vi "Power Output PWM Calibration Warning.vi"(8 "error in (no error)":errorcluster={"status"=FALSE, "code"=0, "source"="WinUtil Master.vi"}, 11 "Message (\"\")":string="The PWM must be calibrated with each execution of this test step.  Spartan always records the instrument calibration state when test sequences are executed.\n\nPlease select one of the following options:\n\n    Calibrate  -  run a calibration on the instrument now\n    Ignore  -  continue without calibration\n    Abort  -  abort this test step\n    Abort All  -  abort the entire sequence") -> (0 "error out":errorcluster={"status"=FALSE, "code"=0, "source"="WinUtil Master.vi"}, 3 "Choice":T1=enum."Calibrate")   [LabVIEW 2011]
uses:
  TypeDefs/Power Output Dialog Response.ctl
panel:
  in  "Abort All":bool
  in  "Abort":bool
  in  "Ignore":bool
  in  "Calibrate":bool
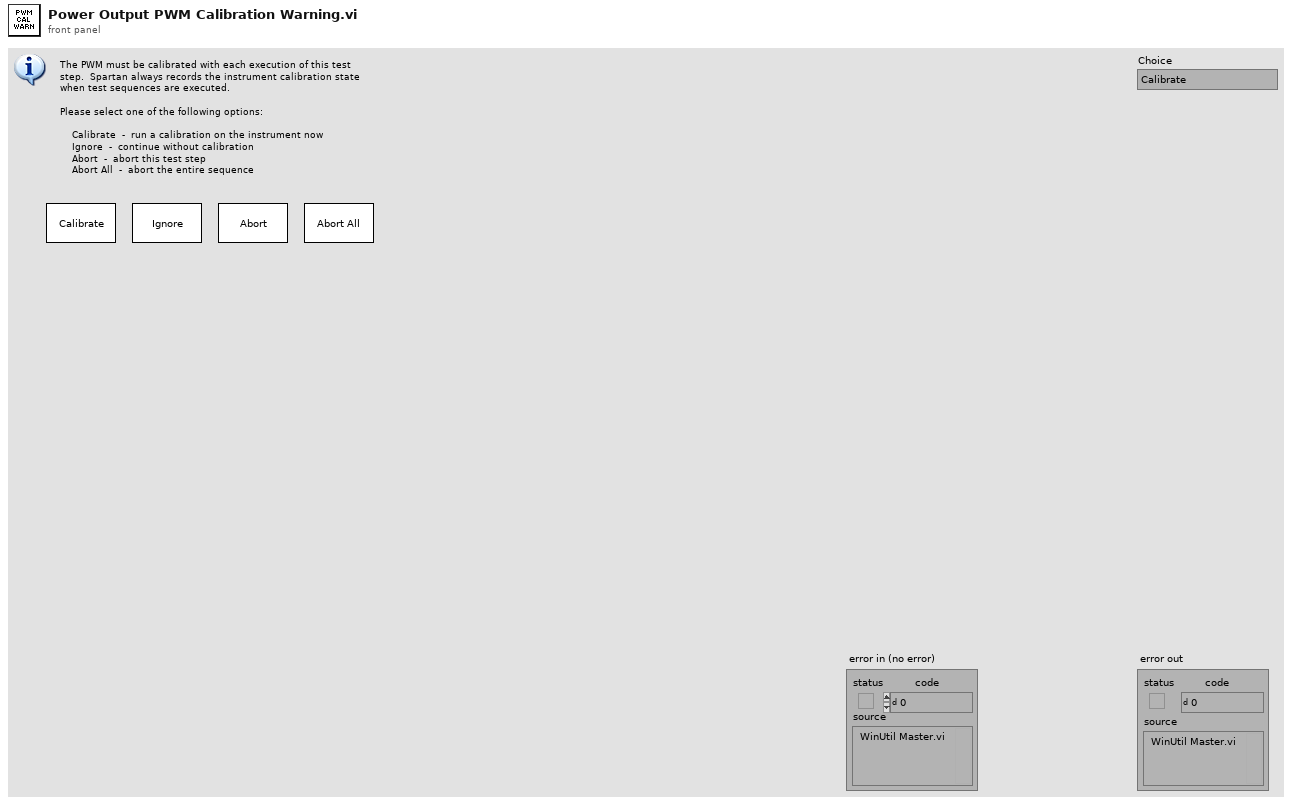
[diagram p1: front panel]
types:
  T1 = typedef "Power Output Dialog Response.ctl" = enum16{"Continue", "Calibrate", "Ignore", "Abort", "Abort All"}
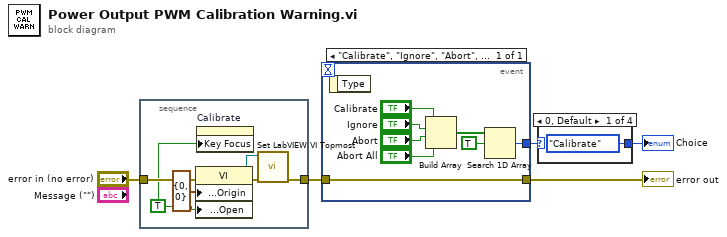
[diagram p0: block diagram]
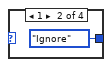
[diagram p2: hidden frame]
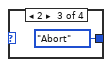
[diagram p3: hidden frame]
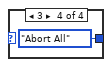
[diagram p4: hidden frame]
diagram:
  n1 = stacked-sequence {
    tunnel: "error in (no error)" -> [w11]
    tunnel: [w8] -> w3
    frame #0 {
      w6 = TRUE ("Front Panel Window:Open")
      n2 = property on="Property Node" class="VI"(error in=w11, "Front Panel Window:Origin"=cluster{"Horizontal":i16, "Vertical":i16} {"Horizontal"=0, "Vertical"=0}, "Front Panel Window:Open"=w6) -> (reference out=w7:refnum<vi>, error out=w9:errorcluster)  [unwired: 1 in]
      n3 = property on="Calibrate" class="Bool"("Key Focus"=w6) -> ()  [unwired: 2 in, 2 out]
      n4 = call "Set LabVIEW VI Topmost.vi"("error in (no error)"=w9, "VI Refnum (null)"=w7) -> ("error out"=w8:errorcluster)  [unwired: 7 in, 2 out]
    }
  }
  n5 = event shown="[0] \"Calibrate\", \"Ignore\", \"Abort\", \"Abort All\": Value Change" {
    selector: _ -> [_]
    dyn-events: _ -> [_]
    timeout: _ -> [_]
    tunnel: w3 -> [w19]
    tunnel: [w19] -> w5
    tunnel: [w13] -> w2
    event "Calibrate", "Ignore", "Abort", "Abort All": Value Change {
      n6 = event-data() -> ()  [unwired: 2 out]
      n7 = Build Array("Calibrate", "Ignore", "Abort", "Abort All") -> (w15:bool[])
      n8 = Search 1D Array(1D array=w15, element=TRUE) -> (index of element=w13:i32)  [unwired: 1 out]
    }
  }
  "error out" <- w5
  n9 = case shown="0, Default" w2 {
    tunnel: [Power_Output_Dialog_Response."Calibrate" ("Action") Power_Output_Dialog_Response."Ignore" ("Action") Power_Output_Dialog_Response."Abort" ("Action") Power_Output_Dialog_Response."Abort All" ("Action")] -> w1
    frame 0, Default {
    }
    frame 1 {
    }
    frame 2 {
    }
    frame 3 {
    }
  }
  "Choice" <- w1
